vi "replaceNodeIn.vi"(8 "error in (no error)":errorcluster, 9 "replaceNodeIn":string, 10 "xmlNodeReplacement":refnum<class "xmlNode.lvclass">, 11 "xmlNode in":refnum<class "xmlNode.lvclass">) -> (0 "error out":errorcluster, 3 "xmlNode out":refnum<class "xmlNode.lvclass">)   [LabVIEW 2011, in "Tools.lvlib" / "xml.lvlib" / "xmlNode.lvclass"]
uses:
  xmlNode.lvclass
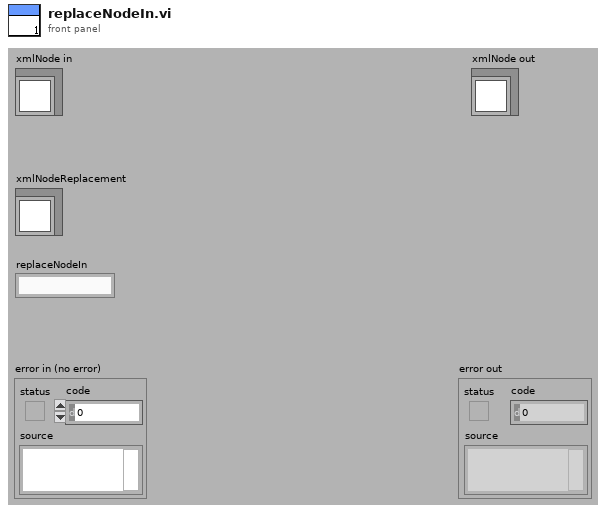
[diagram p1: front panel]
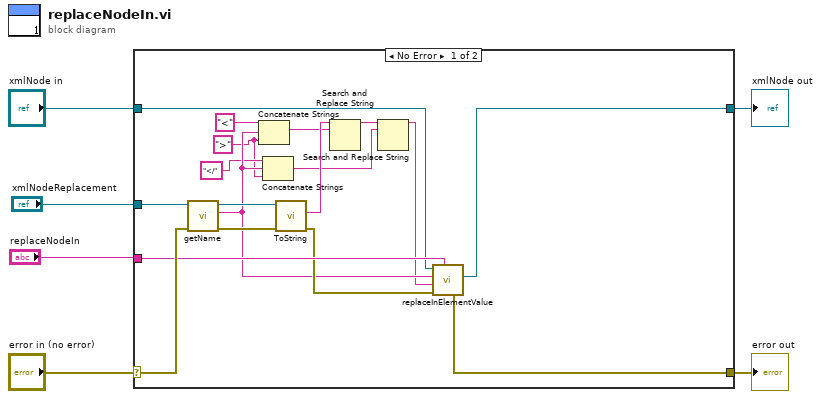
[diagram p0: block diagram]
diagram:
  n1 = case shown="No Error" "error in (no error)" {
    selector: "error in (no error)" -> [w23 w26]
    tunnel: [w16 w26] -> w5
    tunnel: [w17 w25] -> w3
    tunnel: "xmlNode in" -> [w18 w25]
    tunnel: "xmlNodeReplacement" -> [w24 _]
    tunnel: "replaceNodeIn" -> [w20 _]
    frame No Error {
      w7 = ">"
      n2 = call-dynamic "getName.vi"("error in (no error)"=w23, "xmlNode.lvclass in"=w24) -> ("error out"=w21:errorcluster, "name"=w12:string, "xmlNode.lvclass out"=w22:refnum<class "xmlNode.lvclass">)  [unwired: 7 in]
      n3 = Concatenate Strings("<", w12, w7) -> (w13:string)
      n4 = Concatenate Strings("</", w12, w7) -> (w10:string)
      n5 = call-dynamic "ToString.vi"("error in (no error)"=w21, "xmlNode in"=w22) -> ("error out"=w19:errorcluster, "xml"=w15:string)  [unwired: 7 in, 1 out]
      n6 = Search and Replace String(input string=w15, search string=w13) -> (result string=w14:string)  [unwired: 6 in, 3 out]
      n7 = Search and Replace String(input string=w14, search string=w10) -> (result string=w9:string)  [unwired: 6 in, 3 out]
      n8 = call-dynamic "replaceInElementValue.vi"("replaceElementIn"=w20, "error in (no error)"=w19, "replaceWithValue"=w9, "replacementElementName"=w12, "xmlNode in"=w18) -> ("error out"=w16:errorcluster, "replacementxXmlNode"=w17:refnum<class "xmlNode.lvclass">)  [unwired: 4 in, 1 out]
    }
    frame Error {
    }
  }
  "error out" <- w5
  "xmlNode out" <- w3
